vi "Set All Vacuum.vi"(8 "error in":errorcluster, 10 "Channel Array":bool[](array[boolean]), 11 "Gantry Class in":refnum<class "Gantry Class.lvclass">) -> (0 "error out":errorcluster, 3 "Gantry Class out":refnum<class "Gantry Class.lvclass">)   [LabVIEW 2011]
uses:
  Gantry Class/Gantry Class.lvclass
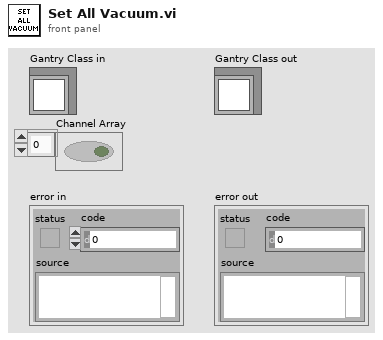
[diagram p1: front panel]
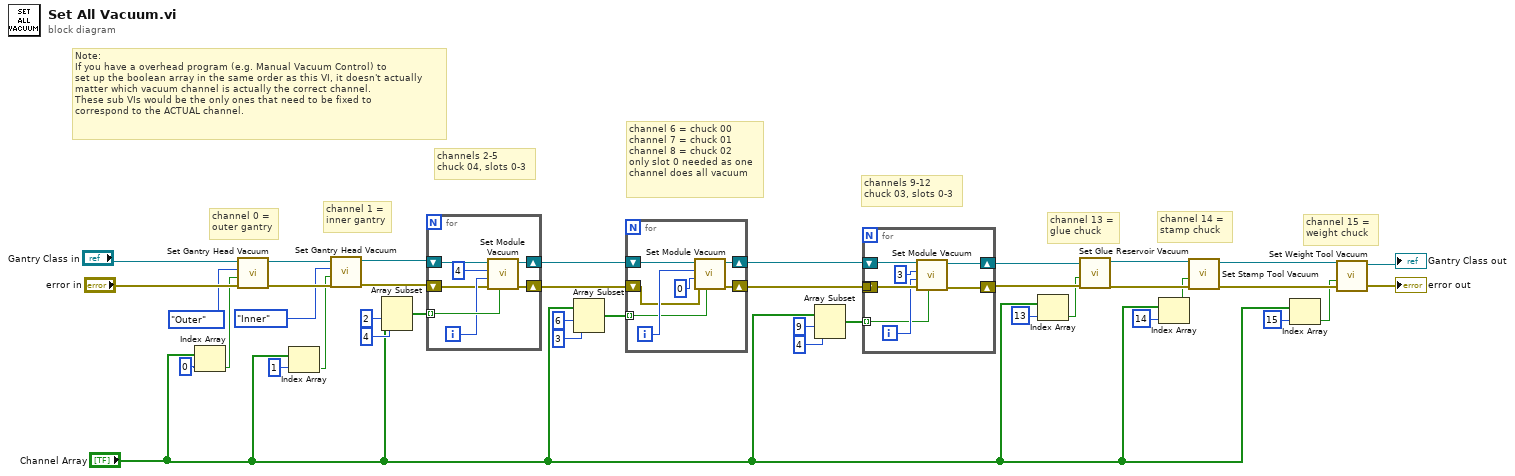
[diagram p0: block diagram]
diagram:
  # "Note:\nIf you have a overhead program (e.g. Manual Vacuum Control) to \nset up the boolean array in the same order as this VI, it doesn't actually\nmatter which vacuum channel is actually the correct channel.  \nThese sub VIs would be the only ones that need to be fixed to\ncorrespond to the ACTUAL channel."
  # "channel 15 =\nweight chuck"
  # "channel 14 = \nstamp chuck"
  # "channel 13 =\nglue chuck"
  # "channels 9-12\nchuck 03, slots 0-3"
  # "channel 6 = chuck 00\nchannel 7 = chuck 01\nchannel 8 = chuck 02\nonly slot 0 needed as one\nchannel does all vacuum"
  # "channels 2-5\nchuck 04, slots 0-3"
  # "channel 1 =\ninner gantry"
  # "channel 0 =\nouter gantry"
  n1 = Index Array(array="Channel Array", index=0) -> (element=w34:bool)
  n2 = call-dynamic "Set Gantry Head Vacuum.vi"("error in (no error)"="error in", "On/Off"=w34, "Inner/Outer"=enum16{"Outer", "Inner"}."Outer", "Gantry Class in"="Gantry Class in") -> ("error out"=w38:errorcluster, "Gantry Class out"=w35:refnum<class "Gantry Class.lvclass">)  [unwired: 6 in]
  n3 = Index Array(array="Channel Array", index=1) -> (element=w31:bool)
  n4 = call-dynamic "Set Gantry Head Vacuum.vi"("error in (no error)"=w38, "On/Off"=w31, "Inner/Outer"=enum16{"Outer", "Inner"}."Inner", "Gantry Class in"=w35) -> ("error out"=w26:errorcluster, "Gantry Class out"=w27:refnum<class "Gantry Class.lvclass">)  [unwired: 6 in]
  n5 = Array Subset(array="Channel Array", index=2, length=4) -> (w29:bool[])
  n6 = for {
    tunnel: w29 -> [w46] mode=indexing
    shift-right: [w43] -> w22
    shift-left: w27 -> [w44]
    shift-right: [w41] -> w21
    shift-left: w26 -> [w42]
    i -> [w45]
    n7 = call-dynamic "Set Module Vacuum.vi"("On/Off"=w46, "error in"=w42, "Slot Number"=w45, "Chuck Number"=4, "Gantry in"=w44) -> ("error out"=w41:errorcluster, "Gantry out"=w43:refnum<class "Gantry Class.lvclass">)  [unwired: 5 in]
  }
  n8 = Array Subset(array="Channel Array", index=6, length=3) -> (w23:bool[])
  n9 = for {
    tunnel: w23 -> [w52] mode=indexing
    shift-right: [w50] -> w20
    shift-left: w22 -> [w51]
    shift-right: [w48] -> w19
    shift-left: w21 -> [w49]
    i -> [w53]
    n10 = call-dynamic "Set Module Vacuum.vi"("On/Off"=w52, "error in"=w49, "Slot Number"=0, "Chuck Number"=w53, "Gantry in"=w51) -> ("error out"=w48:errorcluster, "Gantry out"=w50:refnum<class "Gantry Class.lvclass">)  [unwired: 5 in]
  }
  n11 = Array Subset(array="Channel Array", index=9, length=4) -> (w16:bool[])
  n12 = for {
    tunnel: w19 -> [w60]
    shift-right: [w59] -> w13
    shift-left: w20 -> [w61]
    shift-right: [w58] -> w12
    shift-left: _ -> [_]
    tunnel: w16 -> [w56] mode=indexing
    i -> [w57]
    n13 = call-dynamic "Set Module Vacuum.vi"("On/Off"=w56, "error in"=w60, "Slot Number"=w57, "Chuck Number"=3, "Gantry in"=w61) -> ("error out"=w58:errorcluster, "Gantry out"=w59:refnum<class "Gantry Class.lvclass">)  [unwired: 5 in]
  }
  n14 = Index Array(array="Channel Array", index=13) -> (element=w11:bool)
  n15 = call-dynamic "Set Glue Reservoir Vacuum.vi"("error in (no error)"=w12, "On/Off"=w11, "Gantry Class in"=w13) -> ("error out"=w8:errorcluster, "Gantry Class out"=w9:refnum<class "Gantry Class.lvclass">)  [unwired: 7 in]
  n16 = Index Array(array="Channel Array", index=14) -> (element=w7:bool)
  n17 = call-dynamic "Set Stamp Tool Vacuum.vi"("error in"=w8, "On/Off"=w7, "Gantry in"=w9) -> ("error out"=w4:errorcluster, "Gantry out"=w5:refnum<class "Gantry Class.lvclass">)  [unwired: 7 in]
  n18 = Index Array(array="Channel Array", index=15) -> (element=w2:bool)
  n19 = call-dynamic "Set Weight Tool Vacuum.vi"("error in"=w4, "On/Off"=w2, "Gantry in"=w5) -> ("error out"=→"error out":errorcluster, "Gantry out"=→"Gantry Class out":refnum<class "Gantry Class.lvclass">)  [unwired: 7 in]
